vi "tcpConnectionID.vi"(7 "function":enum16{"read", "write"}(ring)=enum."write", 10 "connection ID":refnum<k5>) -> (2 "connection ID out":refnum<k5>)   [LabVIEW 2018, in "TcpServer.lvclass"]
doc: "FGV to store the tcp connection ID to be shared between the read tcp loop and the sender loop, inside of Tcp Server subVI."
uses:
  TcpServer.lvclass
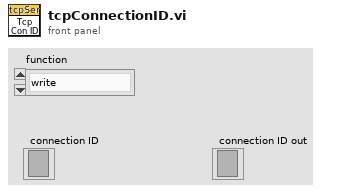
[diagram p1: front panel]
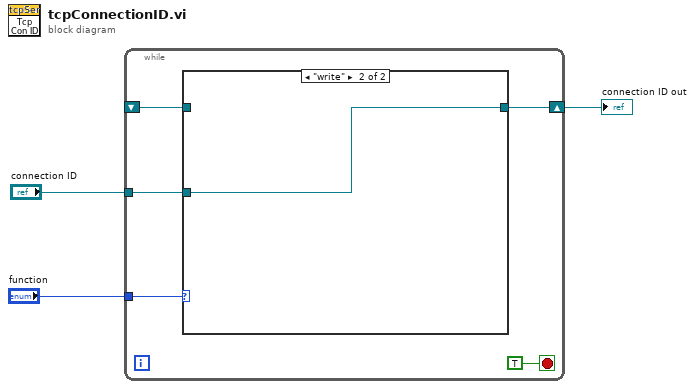
[diagram p0: block diagram]
diagram:
  n1 = while {
    tunnel: "function" -> [w7]
    tunnel: "connection ID" -> [w6]
    shift-right: [w5] -> w1
    shift-left: _ -> [w4]
    stop <- TRUE stop-if-true
    n2 = case shown="\"write\"" w7 {
      tunnel: w6 -> [_ w10]
      tunnel: [w9 w10] -> w5
      tunnel: w4 -> [w9 _]
      frame "read", Default {
      }
      frame "write" {
      }
    }
  }
  "connection ID out" <- w1
